vi "NART Constants.vi"() -> ()   [LabVIEW 2012]
panel:
  in  "Op Set Measured Power":string="cal"
  in  "Request Save Cal":string="Commit Memory=OTP"
  in  "Request Exit":string="Exit"
  in  "Op Aborted Ack":string="OFF"
  in  "Request Op Abort":string="Stop"
  in  "Request Op Initiate":string="Start"
  in  "Op Finished Ack":string="OFF"
  in  "Cmd Completed Ack":string="DONE"
  in  "Error Ack":string="ERROR"
  in  "Op Initiated Ack":string="ON"
  in  "Committed Ack":string="OK"
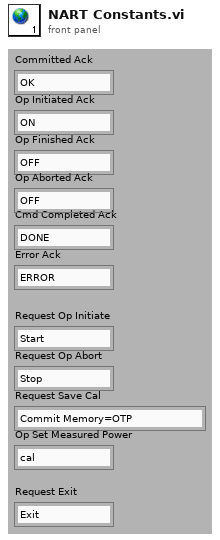
[diagram p1: front panel]
diagram:
